vi "HIOKI PW3390 Conf Operation.vi"(0 "VISA Resource":refnum<visa-resource-name>, 1 "Set/Query (F: Set)":bool, 5 "Operation (0: TYPE1)":enum16{"TYPE1", "TYPE2"}(ring), 11 "error in (no error)":errorcluster, 12 "OPC query (T: ON)":bool=TRUE, 13 "Error Out (F: Off)":bool) -> (4 "VISA Resource out":refnum<visa-resource-name>, 6 "Operation out":enum16{"TYPE1", "TYPE2"}(ring), 15 "error out":errorcluster)   [LabVIEW 2009]
doc: "Sets and reads the formulas of three-phase power.\n\nSet/Query\n Set: Send the setting commands for the device.\n Query: Query the setting of the device.\n\nOperation\n Sets the formulas of three-phase power.\n\n<B>Note</B>\nThis is valid only when the wiring is \"3P3W3M, 1P2W\"."
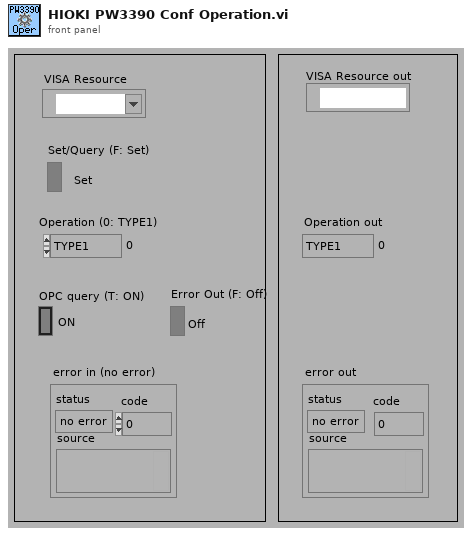
[diagram p1: front panel]
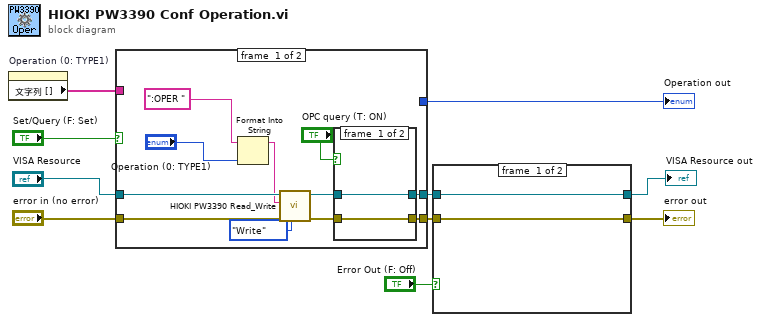
[diagram p0: block diagram]
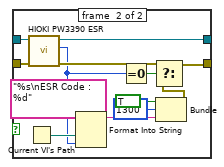
[diagram p2: hidden frame]
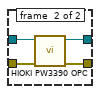
[diagram p3: hidden frame]
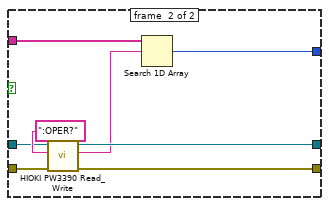
[diagram p4: hidden frame]
diagram:
  n1 = property on="Operation (0: TYPE1)" class="Enum （指定）"() -> ("文字列 []"=w3:string[])  [unwired: 2 in, 2 out]
  n2 = case shown="FALSE" "Set/Query (F: Set)" {
    tunnel: "error in (no error)" -> [w19 w31]
    tunnel: [w12 w34] -> w6
    tunnel: "VISA Resource" -> [w20 w32]
    tunnel: [w11 w33] -> w5
    tunnel: [_ w29] -> w8
    tunnel: w3 -> [_ w30]
    frame #0 {
      n3 = Format Into String(initial string=":OPER ", "Operation (0: TYPE1)") -> (resulting string=w17:string)  [unwired: 2 in, 1 out]
      n4 = call <instrlib>:"HIOKI PW3390 Read_Write.vi"("Read/Write"=enum16{"Read", "Write"}."Write", "error in (no error)"=w19, "data in"=w17, "VISA Resource"=w20) -> ("error out"=w13:errorcluster, "VISA Resource out"=w14:refnum<visa-resource-name>)  [unwired: 5 in, 1 out]
      n5 = case shown="TRUE" "OPC query (T: ON)" {
        tunnel: [w22 w27] -> w11
        tunnel: w14 -> [w22 w25]
        tunnel: w13 -> [w23 w24]
        tunnel: [w23 w26] -> w12
        frame #0 {
        }
        frame #1 {
          n6 = call <instrlib>:"HIOKI PW3390 OPC.vi"("error in (no error)"=w24, "VISA Resource"=w25) -> ("error out"=w26:errorcluster, "VISA Resource out"=w27:refnum<visa-resource-name>)  [unwired: 7 in, 1 out]
        }
      }
    }
    frame #1 {
      n7 = call <instrlib>:"HIOKI PW3390 Read_Write.vi"("error in (no error)"=w31, "data in"=":OPER?", "VISA Resource"=w32) -> ("error out"=w34:errorcluster, "data out"=w28:string, "VISA Resource out"=w33:refnum<visa-resource-name>)  [unwired: 6 in]
      n8 = Search 1D Array(1D array=w30, element=w28) -> (index of element=w29:i32)  [unwired: 1 in]
    }
  }
  "Operation out" <- w8
  n9 = case shown="TRUE" "Error Out (F: Off)" {
    tunnel: w5 -> [w37 w50]
    tunnel: w6 -> [w36 w49]
    tunnel: [w36 w39] -> w4
    tunnel: [w37 w48] -> w1
    frame #0 {
    }
    frame #1 {
      n10 = Current VI's Path() -> (path=w46:path)
      n11 = call <instrlib>:"HIOKI PW3390 ESR.vi"("error in (no error)"=w49, "VISA Resource"=w50) -> ("error out"=w40:errorcluster, "Output Value"=w38:u8, "VISA Resource out"=w48:refnum<visa-resource-name>)  [unwired: 6 in, 1 out]
      n12 = Format Into String(format string="%s\nESR Code : %d", w46, w38) -> (resulting string=w42:string)  [unwired: 2 in, 1 out]
      n13 = Equal To 0?(x=w38) -> (x = 0?=w47:bool)
      n14 = Bundle("status"=TRUE, "code"=1300, w42) -> (w41:cluster{"status":bool, "code":i32, string})  [unwired: 1 in]
      n15 = Select(t=w40, s=w47, f=w41) -> (s? t:f=w39:errorcluster)
    }
  }
  "error out" <- w4
  "VISA Resource out" <- w1
